vi "ReInit All Controls Value.vi"(8 "错误输入（无错误）":errorcluster, 11 "VI Ref":refnum<vi>) -> (0 "错误输出":errorcluster, 3 "引用输出":refnum<vi>)   [LabVIEW 2011]
uses:
  VIRef.lvlib
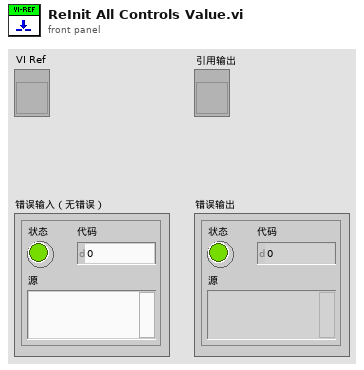
[diagram p1: front panel]
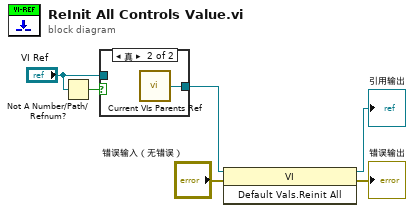
[diagram p0: block diagram]
diagram:
  n1 = Not A Number/Path/Refnum?(number/path/refnum="VI Ref") -> (NaN/Path/Refnum?=w6:bool)
  n2 = case shown="真" w6 {
    tunnel: [w7 w8] -> w4
    tunnel: "VI Ref" -> [w7 _]
    frame False {
    }
    frame True {
      n3 = call "Current VIs Parents Ref.vi"() -> ("Calling VI's Reference"=w8:refnum<vi>)  [unwired: 2 in]
    }
  }
  n4 = invoke class="VI" method="Default Vals.Reinit All"(reference=w4, error in="错误输入（无错误）") -> (reference out=→"引用输出":refnum<vi>, error out=→"错误输出":errorcluster)  [unwired: 1 in, 1 out]
